vi "WrtTempFile.vi"(3 "Trigger Times":dbl[](array[numeric]) format="%.2f", 4 "Input Path":path) -> ()   [LabVIEW 2018]
uses:
  <vilib>/Utility/file.llb/Write Delimited Spreadsheet (DBL).vi
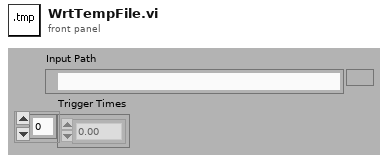
[diagram p1: front panel]
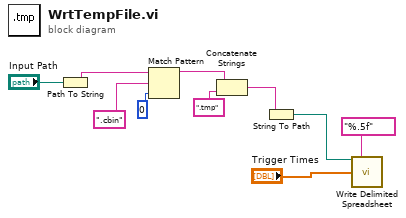
[diagram p0: block diagram]
diagram:
  n1 = Path To String(path="Input Path") -> (string=w10:string)
  n2 = Match Pattern(string=w10, regular expression=".cbin", offset (0)=0) -> (before substring=w7:string)  [unwired: 3 out]
  n3 = Concatenate Strings(w7, ".tmp" ("Substring")) -> (w5:string)
  n4 = String To Path(string=w5) -> (path=w4:path)
  n5 = call-poly <vilib>:"Write Delimited Spreadsheet.vi"("file path (dialog if empty)"=w4, "format (%.3f)"="%.5f", "1D data"="Trigger Times") -> ()  [unwired: 11 in, 2 out]
